vi "Read SET errors.vi"(8 "error in (no error)":errorcluster, 11 "Simulated Camera in":refnum<class "Simulated Camera.lvclass">) -> (0 "error out":errorcluster, 2 "SET errors":T1, 3 "Simulated Camera out":refnum<class "Simulated Camera.lvclass">)   [LabVIEW 2018, in "Simulated Camera.lvclass"]
uses:
  Simulated Camera.lvclass
  Simulated Camera.lvclass/Simulated Camera.ctl
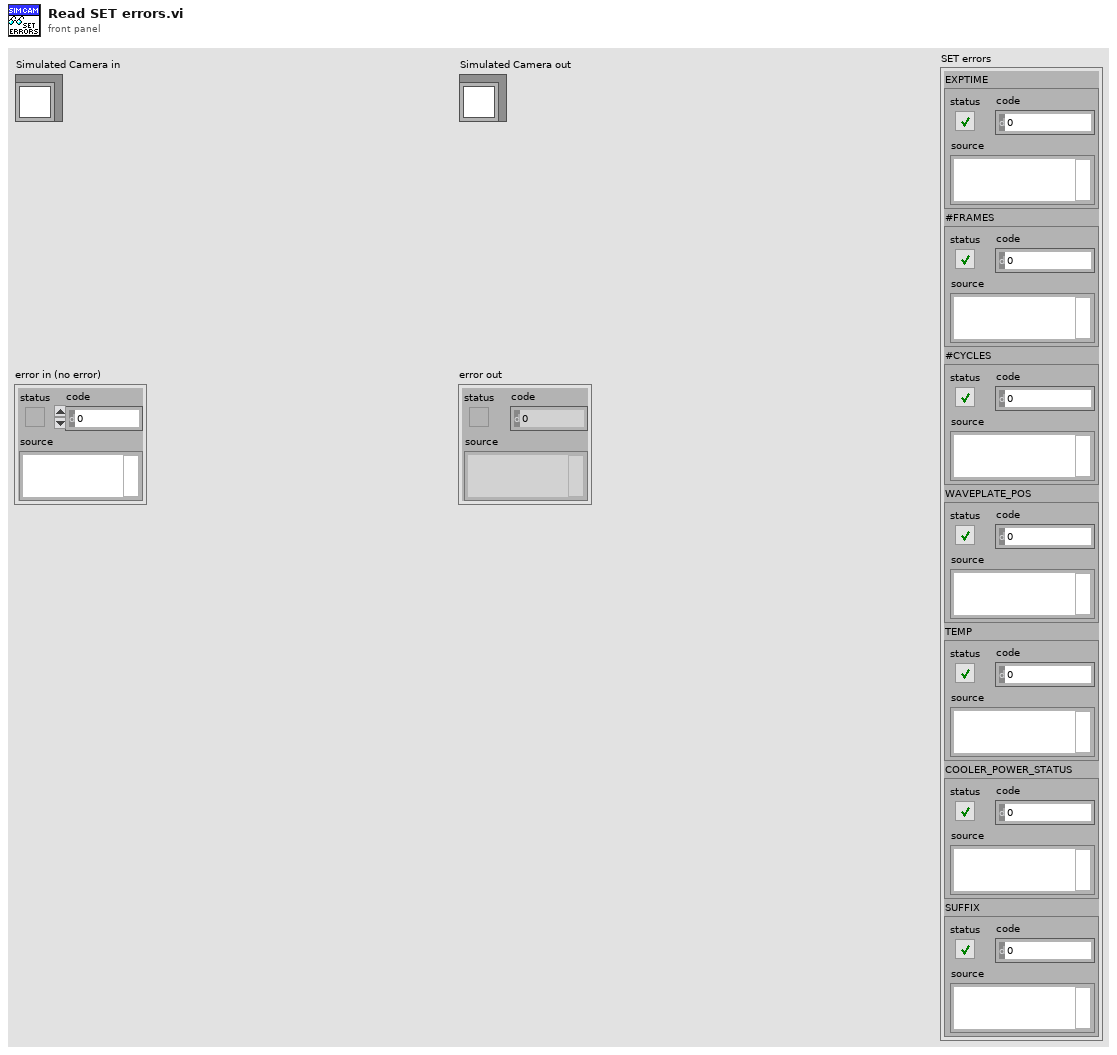
[diagram p1: front panel]
types:
  T1 = cluster{"EXPTIME":errorcluster, "#FRAMES":errorcluster, "#CYCLES":errorcluster, "WAVEPLATE_POS":errorcluster, "TEMP":errorcluster, "COOLER_POWER_STATUS":errorcluster, "SUFFIX":errorcluster}
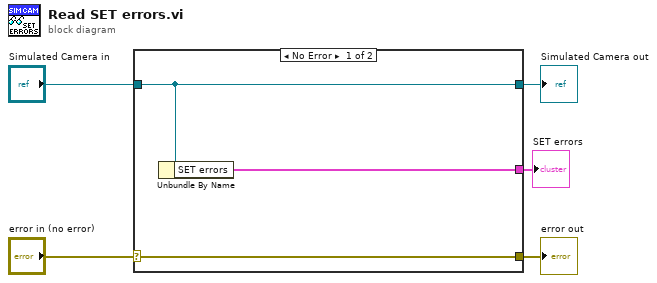
[diagram p0: block diagram]
diagram:
  n1 = case shown="No Error" "error in (no error)" {
    selector: "error in (no error)" -> [w8 w9]
    tunnel: [w8 w9] -> w4
    tunnel: [w7 w10] -> w2
    tunnel: "Simulated Camera in" -> [w7 w10]
    tunnel: [w6 _] -> w1
    frame No Error {
      n2 = Unbundle By Name(w7) -> ("SET errors"=w6:T1)
    }
    frame Error {
    }
  }
  "error out" <- w4
  "Simulated Camera out" <- w2
  "SET errors" <- w1
